vi "GetLogDirectory.vi"(8 "error in (no error)":errorcluster) -> (0 "error out":errorcluster, 3 "log dir":path)   [LabVIEW 2017, in "GlobalConfiguration.lvlib"]
doc: "Returns the path of the directory where the device stores configuration JSON files from the server."
uses:
  <vilib>/addons/InsightCM/Utilities/GlobalConfiguration/GlobalConfiguration.lvlib
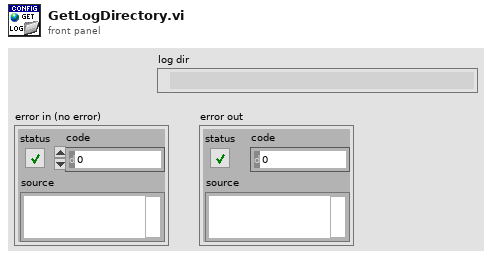
[diagram p1: front panel]
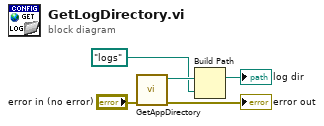
[diagram p0: block diagram]
diagram:
  n1 = call <vilib>:"GetAppDirectory.vi"("error in (no error)"="error in (no error)") -> ("error out"=→"error out":errorcluster, "application directory"=w3:path)  [unwired: 9 in]
  n2 = Build Path(base path=w3, name or relative path=path "logs" ("Log directory")) -> (appended path=→"log dir":path)
